vi "Destroy.vi"(8 "Error In":errorcluster, 11 "Context":refnum<class "Context.lvclass">) -> (0 "Error Out":errorcluster)   [LabVIEW 2018, in "Toolkit.lvlib" / "Data.lvlib" / "Context.lvclass"]
uses:
  Context.lvclass
  Context.lvclass/Context.ctl
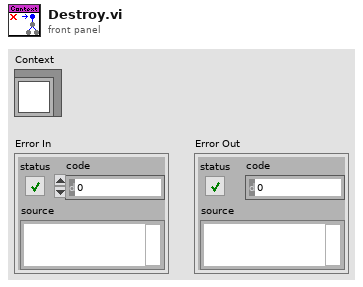
[diagram p1: front panel]
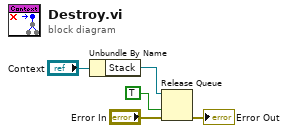
[diagram p0: block diagram]
diagram:
  n1 = Unbundle By Name("Context") -> ("Stack"=w4:refnum<queue>)
  n2 = Release Queue(queue=w4, force destroy? (F)=TRUE, error in (no error)="Error In") -> (error out=→"Error Out":errorcluster)  [unwired: 2 out]
